vi "Configure Trigger.vi"(4 "Slope (0: Positive)":i32(ring) items=["Positive", "Negative"], 5 "Delay Seconds (0 s)":dbl, 6 "Count Number (1)":i32=1, 7 "Timer Value (1 us)":dbl=1e-06, 8 "error in (no error)":errorcluster, 9 "Trigger Source (0: Immediate)":i32(ring) items=["Immediate", "External", "Timer", "Bus"], 10 "Channel (1: 1)":i32(ring)=1 items=["1"=1, "2"=2], 11 "VISA resource name":refnum<visa-resource-name>) -> (0 "error out":errorcluster, 3 "VISA resource name out":refnum<visa-resource-name>)   [LabVIEW 2013, in "AWG.lvlib" / "Agilent 3352X Series.lvlib"]
doc: "Configures the trigger source,count,delay and slop for triggering arbitrary sequence, sweep, list, or burst.\n\n<B>Note</B>: \nThis VI does not check the instrument status."
uses:
  Agilent 3352X Series.lvlib
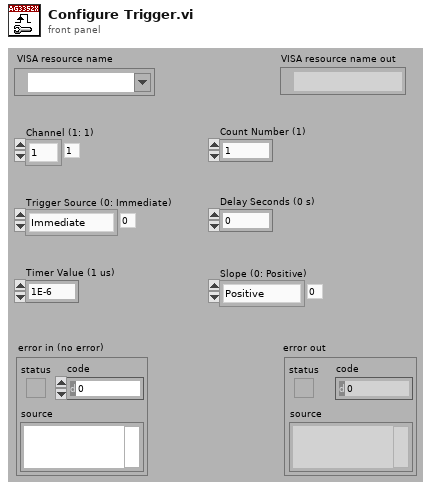
[diagram p1: front panel]
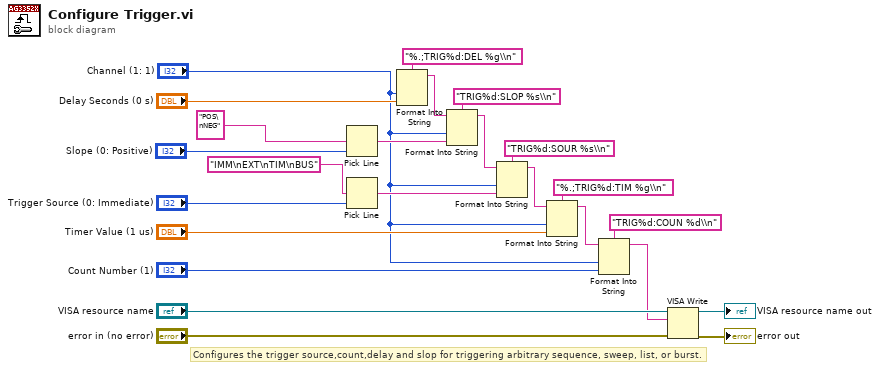
[diagram p0: block diagram]
diagram:
  # "Configures the trigger source,count,delay and slop for triggering arbitrary sequence, sweep, list, or burst."
  n1 = Pick Line(multi-line string="POS\nNEG", line index="Slope (0: Positive)") -> (output string=w9:string)  [unwired: 1 out]
  n2 = Pick Line(multi-line string="IMM\nEXT\nTIM\nBUS", line index="Trigger Source (0: Immediate)") -> (output string=w7:string)  [unwired: 1 out]
  n3 = Format Into String(format string="%.;TRIG%d:DEL %g\\n", "Channel (1: 1)", "Delay Seconds (0 s)") -> (resulting string=w22:string)  [unwired: 2 in, 1 out]
  n4 = Format Into String(format string="TRIG%d:SLOP %s\\n", initial string=w22, "Channel (1: 1)", w9) -> (resulting string=w20:string)  [unwired: 1 in, 1 out]
  n5 = Format Into String(format string="TRIG%d:SOUR %s\\n", initial string=w20, "Channel (1: 1)", w7) -> (resulting string=w18:string)  [unwired: 1 in, 1 out]
  n6 = Format Into String(format string="%.;TRIG%d:TIM %g\\n", initial string=w18, "Channel (1: 1)", "Timer Value (1 us)") -> (resulting string=w4:string)  [unwired: 1 in, 1 out]
  n7 = Format Into String(format string="TRIG%d:COUN %d\\n", initial string=w4, "Channel (1: 1)", "Count Number (1)") -> (resulting string=w3:string)  [unwired: 1 in, 1 out]
  n8 = VISA Write(VISA resource name="VISA resource name", write buffer=w3, error in (no error)="error in (no error)") -> (VISA resource name out=→"VISA resource name out":refnum<visa-resource-name>, error out=→"error out":errorcluster)  [unwired: 1 out]
